vi "Camera Contoller ID CC.vi"(8 "error in (no error)":errorcluster, 10 "Camera Controller ID":i32, 11 "Camera Controller in":refnum<class "Camera Controller.lvclass">) -> (0 "error out":errorcluster, 3 "Camera Controller out":refnum<class "Camera Controller.lvclass">)   [LabVIEW 2019, in "Camera Controller.lvlib" / "Camera Controller.lvclass"]
uses:
  Camera Controller.lvclass
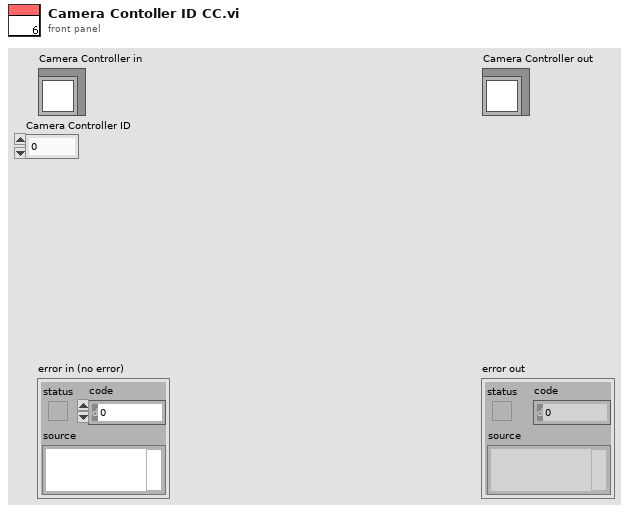
[diagram p1: front panel]
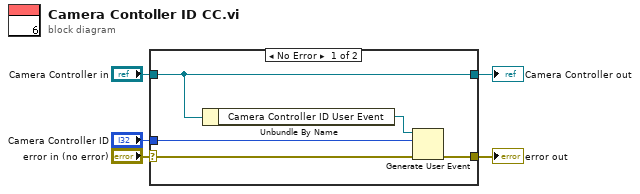
[diagram p0: block diagram]
diagram:
  n1 = case shown="No Error" "error in (no error)" {
    selector: "error in (no error)" -> [w8 w12]
    tunnel: [w7 w12] -> w4
    tunnel: [w6 w11] -> w2
    tunnel: "Camera Controller in" -> [w6 w11]
    tunnel: "Camera Controller ID" -> [w9 _]
    frame No Error {
      n2 = Unbundle By Name(w6) -> ("Camera Controller ID User Event"=w10:refnum<user-event>)
      n3 = Generate User Event(user event=w10, event data cluster=w9, error in=w8) -> (error out=w7:errorcluster)  [unwired: 1 in, 1 out]
    }
    frame Error {
    }
  }
  "error out" <- w4
  "Camera Controller out" <- w2
